vi "VI-tree.vi"() -> ()   [LabVIEW 2013]
doc: "Representation of the main module functions and their relationships/interactions.\nAdditional emphasis on functions and definitions that should be modified by the integrator to the specific use case."
uses:
  SC-Client.lvclass
  Supported-messages.ctl
  Supported-actions.ctl
  Supported-modules.ctl
panel:
  in  "Module type":T1
  in  "Action":T2
  in  "Message":T3
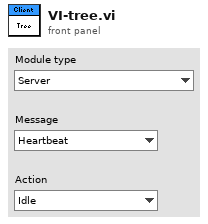
[diagram p1: front panel]
types:
  T1 = typedef "SLMControl.lvlib/SC-Client.lvclass/Supported-modules.ctl" = enum16{"Server", "All", "SLMControl", "PowderDeposition", "StrategyParser", "CameraVision", "MaterialCharacterization", "StatusMonitor", "SLMSimulation", "LaserCharacterization"}
  T2 = typedef "SLMControl.lvlib/SC-Client.lvclass/Supported-actions.ctl" = enum16{"Idle", "Initialize", "Load settings", "Load file", "Activate", "Start", "Pause", "Stop", "Repeat", "Reset", "Exit"}
  T3 = typedef "SLMControl.lvlib/SC-Client.lvclass/Supported-messages.ctl" = enum16{"Heartbeat", "Error", "Start client", "Client stopped", "Action", "Query status", "Send status", "Get clients"}
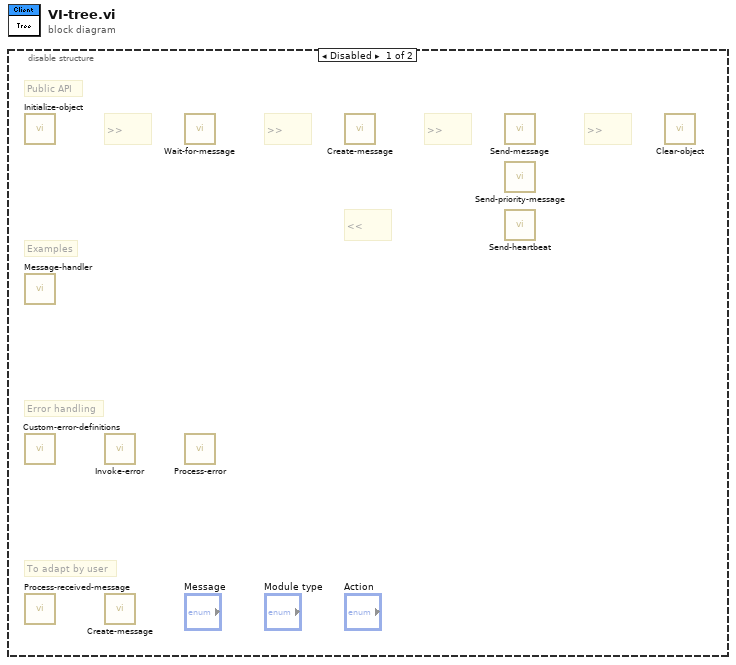
[diagram p0: block diagram]
diagram:
  n1 = disable-structure shown="Disabled" {
    frame Disabled {
      # ">>"
      # "To adapt by user"
      # "Error handling"
      # "<<"
      # "Examples"
      # "Public API"
      # ">>"
      # ">>"
      # ">>"
      n2 = call "Initialize-object.vi"() -> ()  [unwired: 10 in, 2 out]
      n3 = call "Message-handler.vi"() -> ()  [unwired: 10 in, 2 out]
      n4 = call "Custom-error-definitions.vi"() -> ()  [unwired: 9 in, 3 out]
      n5 = call "Process-received-message.vi"() -> ()  [unwired: 9 in, 3 out]
      n6 = call "Invoke-error.vi"() -> ()  [unwired: 11 in, 1 out]
      n7 = call "Create-message.vi"() -> ()  [unwired: 10 in, 2 out]
      n8 = call "Wait-for-message.vi"() -> ()  [unwired: 8 in, 4 out]
      n9 = call "Process-error.vi"() -> ()  [unwired: 10 in, 2 out]
      n10 = call "Create-message.vi"() -> ()  [unwired: 10 in, 2 out]
      n11 = call "Send-message.vi"() -> ()  [unwired: 10 in, 2 out]
      n12 = call "Send-priority-message.vi"() -> ()  [unwired: 10 in, 2 out]
      n13 = call "Send-heartbeat.vi"() -> ()  [unwired: 10 in, 2 out]
      n14 = call "Clear-object.vi"() -> ()  [unwired: 10 in, 2 out]
    }
    frame Enabled {
    }
  }
